vi "BurstModeCompleteRoutedMessage_Name.vi"() -> (1 "message name":string="BurstMode.BurstModeComplete")   [LabVIEW 2017, in "BurstMode.lvlib"]
uses:
  <vilib>/addons/InsightCM/Devices/Shared/Cms/CmsBurstMode/BurstMode.lvlib
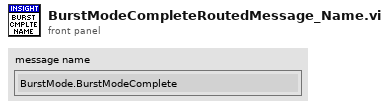
[diagram p1: front panel]
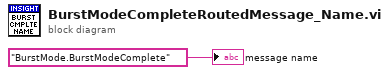
[diagram p0: block diagram]
diagram:
  "message name" <- "BurstMode.BurstModeComplete" ("ProcessName")
